vi "Climb Loop.vi"(10 "Extend Power in":dbl, 11 "Y Power":dbl) -> (1 "Unpin?":bool, 2 "Pull Power":dbl, 3 "PTO Engaged?":bool, 5 "Extend Power":dbl)   [LabVIEW 2015]
uses:
  Common Code/Climb Auto State.ctl
  Robot Global Data.vi
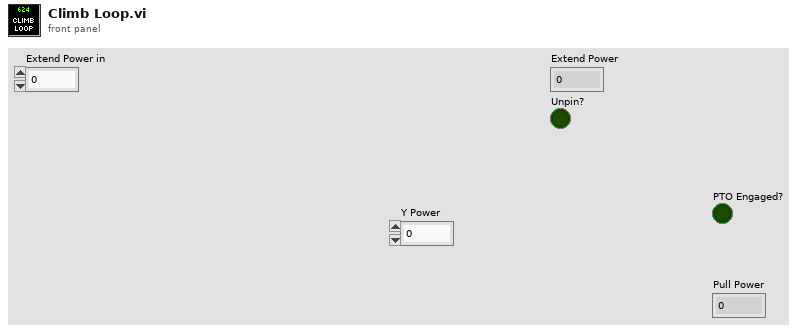
[diagram p1: front panel]
types:
  T1 = typedef "Dashboard Control Data.ctl" = cluster{"Shooter Presets":T2, "Encoder Control":T4, "Steer PID output":cluster{"output high":dbl, "output low":dbl}, " Steer PID gains":cluster{"proportional gain (Kc)":dbl, "integral time (Ti, min)":dbl, "derivative time (Td, min)":dbl}, "Drivetrain Settings":T5, "Vision Packet":T6, "Dashboard Drivetrain Command":T7, "Info/Command Cluster":T9, "Ball Vision Packet":T10, "Intake Presets":T12, "Intake Encoder Control":T14, "Climb Presets":T15, "Goal Output Range":cluster{"output high":dbl, "output low":dbl}, "Enabled Systems":T16, "Auton Presets":T17, "Pressure M":dbl, "Pressure B":dbl}
  T2 = typedef "Shooter Presets.ctl" = cluster{"Batter Shot":T3, "Deep Middle":T3, "Manual Shot":T3, "Left Ticks Per Rotation":dbl, "Right Ticks Per Rotation":dbl, "Low Bar Shot":T3, "Shooter RPM Tolerance":dbl, "IIR Filter Power":dbl, "Trigger Power":dbl, "Fire from Load Delay":i32, "Max Angle":dbl, "Min Angle":dbl, "Angle PID gains":cluster{"P":dbl, "I":dbl, "D":dbl}, "Angle Output":cluster{"output high":dbl, "output low":dbl}, "Shooter Angle Tolerance":dbl, "Vision Shoot x^2":dbl, "Vision Shoot x":dbl, "IR Let Go Timer":dbl, "High Goal Center Height":dbl, "Feed Forward Max Accel":dbl, "Feed Forward Kv":dbl, "Backwards Trigger":dbl, "Shot Finish Delay (ms)":dbl, "Angle Max Current":dbl, "Angle Current Trip Time":dbl, "Intake Angle":dbl, "Vision Shoot c":dbl, "Reset?":bool, "Servo Release Delay":dbl, "Servo Idle Angle":i32, "Servo Hold Angle":i32, "Angle Pot x":dbl, "Angle Pot c":dbl, "Ignore Angle?":bool, "Manual Output?":bool, "Manual Out":dbl, "Max RPM":dbl, "Safty Frist Angle":dbl, "Intake Danger Height":dbl, "Angle Pot B":i32, "Angle Pot M":dbl, "FF Finish RPM":dbl, "RPM PID Right":cluster{"P":dbl, "I":dbl, "D":dbl, "FF":dbl}, "RPM PID Left":cluster{"P":dbl, "I":dbl, "D":dbl, "FF":dbl}, "Backwards RPM":dbl, "Vision RPM":dbl, "Run Wheels Backward Delay":u32, "Cleat Shot":T3}
  T3 = typedef "Shot Presets.ctl" = cluster{"L":dbl, "R":dbl, "A":dbl}
  T4 = typedef "Encoder Control.ctl" = cluster{"Right Tick Constant":dbl, "Left Tick Constant":dbl, "Reset?":bool, "Y Dist":cluster{"PID gains":cluster{"proportional gain (Kc)":dbl, "integral time (Ti, min)":dbl, "derivative time (Td, min)":dbl}}, "Y Stop Thresh":dbl, "Y Stop Speed":dbl}
  T5 = typedef "Drivetrain Settings.ctl" = cluster{"Gyro Tolerance":dbl, "Throttle Ramp (ms)":dbl, "Angular rate compensation":bool, "Throttle to Rate Scale":dbl, "Rate compensation gain":dbl, "Kv":dbl, "Ka":dbl, "Feed Forward P":dbl, "Feed Forward D":dbl, "Goal Vision PID gains":cluster{"proportional gain (Kc)":dbl, "integral time (Ti, min)":dbl, "derivative time (Td, min)":dbl}, "Goal Detection Window":dbl, "Creep Rate":dbl, "Vision Throttle Threshold":dbl, "Min Turn Output":dbl}
  T6 = typedef "Goal Vision Packet.ctl" = cluster{"Distance":dbl, "Center X":dbl, "Center Y":dbl, "Found Target?":bool, "Robot Center":dbl, "Angle":dbl}
  T7 = typedef "Dashboard Drivetrain Command.ctl" = cluster{"Drivetrain Vision":T8}
  T8 = typedef "Drivetrain Vision.ctl" = cluster{"Goal Window":dbl, "Ball Window":dbl}
  T9 = typedef "Ball Tracking Command Cluster.ctl" = cluster{"Distance to Ball":dbl, "Desired Angle":dbl, "Command":enum16{"Turn to Ball", "Turn to Angle", "Get Distance"}, "Pixels from Center":dbl}
  T10 = typedef "Ball Vision Packet.ctl" = cluster{"Ball Detected?":bool, "Distance to Ball":dbl, "Desired Angle":dbl, "Pixels from Center":dbl, "Tracking mode":T11}
  T11 = typedef "Tracking Mode.ctl" = enum16{"Turn to Ball", "Turn to Angle"}
  T12 = typedef "Intake Presets.ctl" = cluster{"Intake Speed":dbl, "Outake Speed":dbl, "Low Height":dbl, "Half Height":dbl, "Full Height":dbl, "Angle Speed":dbl, "Angle Tolerance":dbl, "Encoder Scale":dbl, "Load Height":dbl, "Output Range":T13, "Rotation Power Max/Min":dbl, "MaxCurrent":dbl, "Intake Trip Time":dbl, "Idle Height":dbl, "Max Height":dbl, "Reset Encoders?":bool, "PID gains":cluster{"proportional gain (Kc)":dbl, "integral time (Ti, min)":dbl, "derivative time (Td, min)":dbl}, "Intake Stop Delay":u32}
  T13 = typedef "Drivetrain Output Range.ctl" = cluster{"output high":dbl, "output low":dbl}
  T14 = typedef "IntakeEcoderControl.ctl" = cluster{"Arm Tick Constant":dbl, "Reset?":bool, "Y Dist":cluster{"PID gains":cluster{"proportional gain (Kc)":dbl, "integral time (Ti, min)":dbl, "derivative time (Td, min)":dbl}}, "Y Stop Thresh":dbl, "Y Stop Speed":dbl}
  T15 = typedef "Climb Presets.ctl" = cluster{"Pull Power":dbl, "Time to Hold":dbl, "Extend Power":dbl}
  T16 = typedef "Enabled Systems.ctl" = cluster{"Shoot":bool, "Intake":bool, "DT":bool, "Gyro":bool, "100ms":bool, "US":bool}
  T17 = typedef "Autonomous Presets.ctl" = cluster{"Pitch Limit":dbl, "Roll Limit":dbl, "Ultrasonic Limit":dbl, "Start Position":dbl, "Cross Position":dbl}
  T18 = typedef "Climb Command Cluster.ctl" = cluster{"Climb Mode":T19, "Hold?":bool, "Manual State":T20}
  T19 = typedef "Climb Mode.ctl" = enum16{"Auto", "Semi-Auto", "Manual"}
  T20 = typedef "Climb Manual State.ctl" = cluster{"Release":bool, " PTO Engage":bool, "Extend":bool}
  T21 = typedef "Climb Auto State.ctl" = enum16{"Reach up", "Hold on", "Pull up"}
  T22 = typedef "Climb Status Cluster.ctl" = cluster{"Pull Power":dbl, "Unpin Power":dbl, "PTO Engaged?":bool, "Climb Mode":T19}
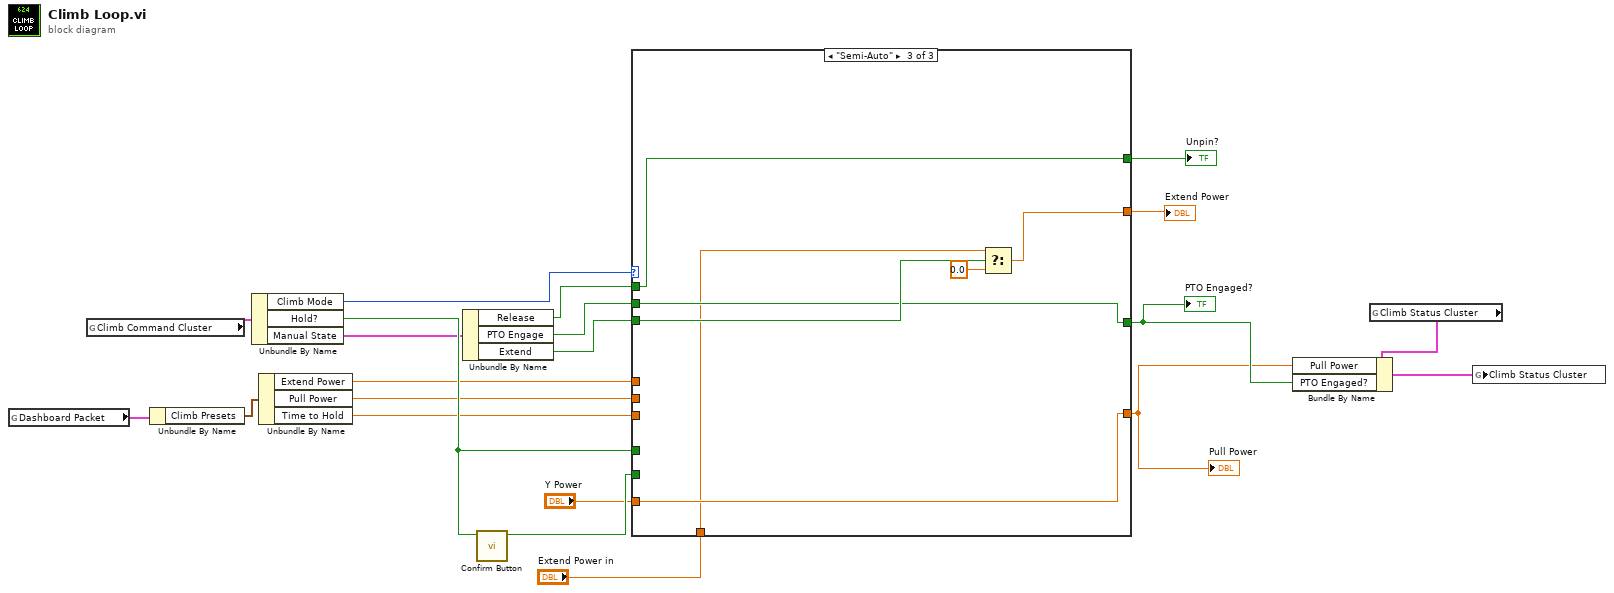
[diagram p0: block diagram]
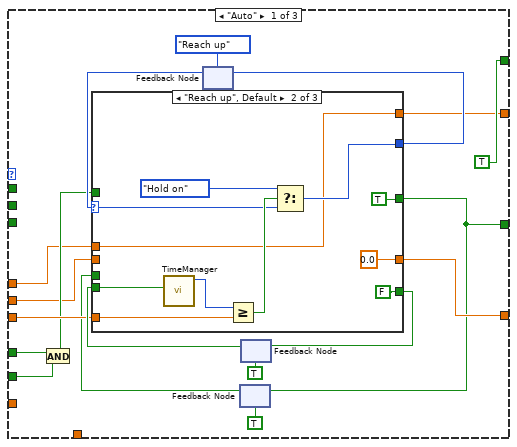
[diagram p2: hidden frame]
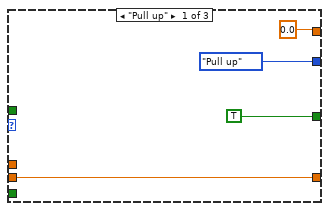
[diagram p3: hidden frame]
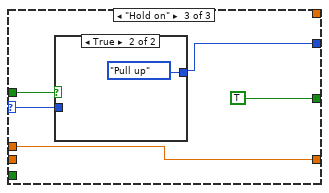
[diagram p4: hidden frame]
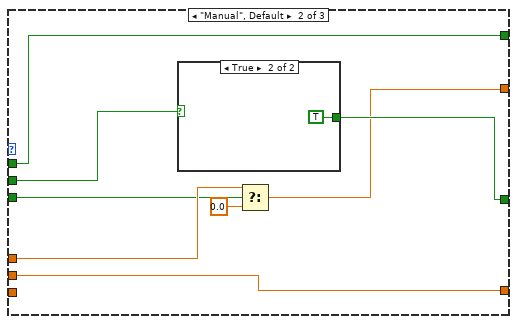
[diagram p6: hidden frame]
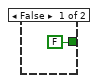
[diagram p7: hidden frame]
diagram:
  n1 = global read "Robot Global Data.vi" "Dashboard Packet"() -> (w17:T1)
  n2 = global read "Robot Global Data.vi" "Climb Command Cluster"() -> (w19:T18)
  n3 = Unbundle By Name(w17) -> ("Climb Presets"=w10:T15)
  n4 = Unbundle By Name(w19) -> ("Climb Mode"=w20:T19, "Hold?"=w18:bool, "Manual State"=w3:T20)
  n5 = Unbundle By Name(w10) -> ("Extend Power"=w13:dbl, "Pull Power"=w12:dbl, "Time to Hold"=w11:dbl)
  n6 = Unbundle By Name(w3) -> ("Release"=w6:bool, "PTO Engage"=w5:bool, "Extend"=w4:bool)
  n7 = call "Confirm Button.vi"("Button"=w18) -> ("Boolean out"=w21:bool)  [unwired: 10 in]
  n8 = case shown="\"Semi-Auto\"" w20 {
    tunnel: w13 -> [w24 w64 _]
    tunnel: [w39 w66 w74] -> w15
    tunnel: [w37 w67 w73] -> w16
    tunnel: w6 -> [_ w69 w75]
    tunnel: w21 -> [w32 _ _]
    tunnel: w5 -> [_ w68 w73]
    tunnel: w12 -> [w22 w66 _]
    tunnel: w18 -> [w33 _ _]
    tunnel: w11 -> [w28 _ _]
    tunnel: [TRUE w69 w75] -> w14
    tunnel: [w23 w65 w76] -> w7
    tunnel: w4 -> [_ w63 w78]
    tunnel: "Y Power" -> [_ _ w74]
    tunnel: "Extend Power in" -> [_ _ w72]
    frame "Auto" {
      n9 = And(x=w33, y=w32) -> (x .and. y?=w26:bool)
      n10 = feedback #1(Climb_Auto_State."Reach up" ("Auto State")) -> (w38:T21)
      n11 = feedback #2(TRUE ("PTO Engage")) -> (w25:bool)
      n12 = feedback #3(TRUE) -> (w31:bool)
      n13 = case shown="\"Reach up\", Default" w38 {
        selector: w38 -> [_ w47 w57]
        tunnel: [w40 0.0 w55] -> w39
        tunnel: [Climb_Auto_State."Pull up" ("Auto State") w54 w56] -> w34
        tunnel: [TRUE ("PTO Engage") TRUE ("PTO Engage") TRUE ("PTO Engage")] -> w37
        tunnel: w25 -> [_ _ _]
        tunnel: w26 -> [_ _ w58]
        tunnel: w24 -> [_ w45 w55]
        tunnel: w28 -> [_ w52 _]
        tunnel: w31 -> [_ w50 _]
        tunnel: [_ FALSE _] -> w30
        tunnel: [0.0 w45 _] -> w23
        tunnel: w22 -> [w40 _ _]
        frame "Pull up" {
        }
        frame "Reach up", Default {
          n14 = call "TimeManager.vi"("Reset?"=w50) -> ("Time Since Reset"=w51:u32)  [unwired: 9 in, 1 out]
          n15 = Greater Or Equal?(x=w51, y=w52) -> (x >= y?=w53:bool)
          n16 = Select(t=Climb_Auto_State."Hold on" ("Auto State"), s=w53, f=w47) -> (s? t:f=w54:T21)
        }
        frame "Hold on" {
          n17 = case shown="True" w58 {
            tunnel: [w60 Climb_Auto_State."Pull up" ("Auto State")] -> w56
            tunnel: w57 -> [w60 _]
            frame False {
            }
            frame True {
            }
          }
        }
      }
      n18 = feedback-in #1(w34) -> ()
      n19 = feedback-in #2(w37) -> ()
      n20 = feedback-in #3(w30) -> ()
    }
    frame "Manual", Default {
      n21 = case shown="True" w68 {
        tunnel: [FALSE TRUE] -> w67
        frame False {
        }
        frame True {
        }
      }
      n22 = Select(t=w64, s=w63, f=0.0) -> (s? t:f=w65:dbl)
    }
    frame "Semi-Auto" {
      n23 = Select(t=w72, s=w78, f=0.0) -> (s? t:f=w76:dbl)
    }
  }
  "Pull Power" <- w15
  "PTO Engaged?" <- w16
  "Extend Power" <- w7
  "Unpin?" <- w14
  n24 = global read "Robot Global Data.vi" "Climb Status Cluster"() -> (w8:T22)
  n25 = Bundle By Name(cluster=w8, "Pull Power"=w15, "PTO Engaged?"=w16) -> (w9:T22)
  n26 = global write "Robot Global Data.vi" "Climb Status Cluster"(w9) -> ()
